vi "QueryDAQHardware.vi"(8 "error in (no error)":errorcluster, 11 "Chassis Reference in":refnum<k39>) -> (0 "error out":errorcluster, 2 "Devices out":string[](array[string]), 3 "Chassis Reference out":refnum<k39>)   [LabVIEW 2027, in "VeriStandTestUtilities.lvlib"]
uses:
  VeriStandTestUtilities.lvlib
  C:/NetCoreDLL/NationalInstruments.VeriStand.SystemDefinitionAPI.dll
  NetCoreDLL/NationalInstruments.VeriStand.SystemDefinitionAPI.dll
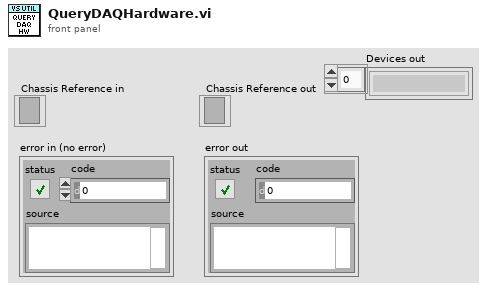
[diagram p1: front panel]
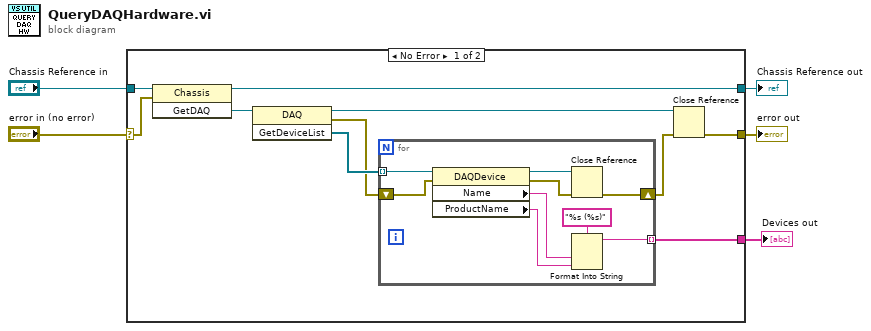
[diagram p0: block diagram]
diagram:
  n1 = case shown="No Error" "error in (no error)" {
    selector: "error in (no error)" -> [w13 w25]
    tunnel: [w7 w25] -> w5
    tunnel: [w15 w26] -> w4
    tunnel: "Chassis Reference in" -> [w14 w26]
    tunnel: [w6 _] -> w1
    frame No Error {
      n2 = invoke class="Chassis" method="GetDAQ"(reference=w14, error in=w13) -> (reference out=w15:refnum<k39>, "GetDAQ"=w12:refnum<k39>)  [unwired: 1 in, 1 out]
      n3 = invoke class="DAQ" method="GetDeviceList"(reference=w12) -> (reference out=w11:refnum<k39>, error out=w9:errorcluster, "GetDeviceList"=w10:refnum<k39>[])  [unwired: 2 in]
      n4 = for {
        tunnel: w10 -> [w23] mode=indexing
        shift-right: [w24] -> w8
        shift-left: w9 -> [w21]
        tunnel: [w17] -> w6 mode=indexing
        n5 = property class="DAQDevice"(reference=w23, error in=w21) -> (reference out=w22:refnum<k39>, error out=w20:errorcluster, "Name"=w19:string, "ProductName"=w18:string)
        n6 = Close Reference(reference=w22, error in (no error)=w20) -> (error out=w24:errorcluster)
        n7 = Format Into String(format string="%s (%s)", w19, w18) -> (resulting string=w17:string)  [unwired: 2 in, 1 out]
      }
      n8 = Close Reference(reference=w11, error in (no error)=w8) -> (error out=w7:errorcluster)
    }
    frame Error {
    }
  }
  "error out" <- w5
  "Chassis Reference out" <- w4
  "Devices out" <- w1
